vi "Add Item to Tree.vi"(6 "Extra Info":string, 7 "Parent Tag":string, 8 "error in (no error)":errorcluster, 9 "Item Name":string, 10 "Item Tag":string, 11 "Tree Ref":refnum<vi>) -> (0 "error out":errorcluster, 1 "Item Name out":string, 2 "Item Tag out":string, 3 "reference out":refnum<vi>)   [LabVIEW 2018]
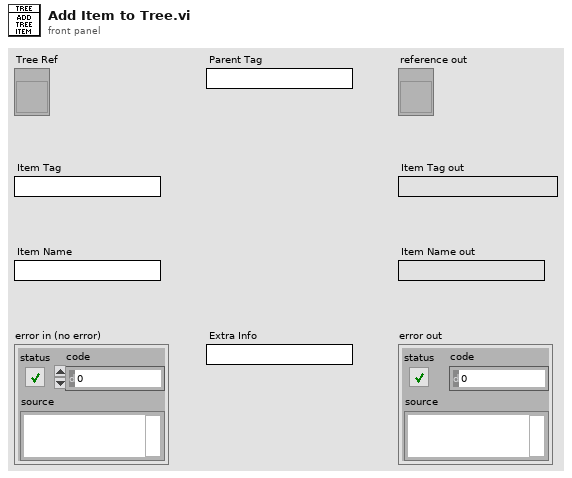
[diagram p1: front panel]
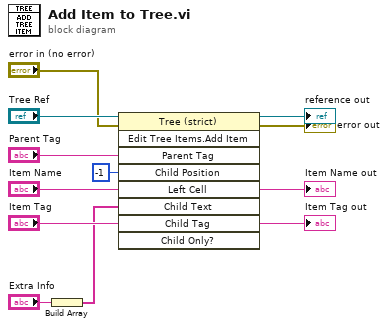
[diagram p0: block diagram]
diagram:
  n1 = Build Array("Extra Info") -> (w1:string[])
  n2 = invoke class="Tree (strict)" method="Edit Tree Items.Add Item"(reference="Tree Ref", error in="error in (no error)", "Parent Tag"="Parent Tag", "Child Position"=-1, "Left Cell"="Item Name", "Child Text"=w1, "Child Tag"="Item Tag") -> (reference out=→"reference out":refnum<vi>, error out=→"error out":errorcluster)  [unwired: 2 in, 7 out]
  "Item Tag out" <- "Item Tag"
  "Item Name out" <- "Item Name"
